vi "Range.vi"(9 "Range":dbl, 10 "Input":dbl, 11 "In Range of":dbl) -> (3 "In Range?":bool)   [LabVIEW 2014]
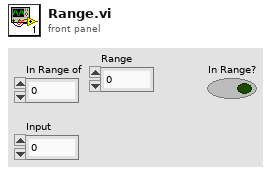
[diagram p1: front panel]
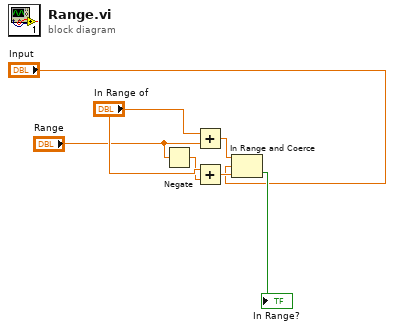
[diagram p0: block diagram]
diagram:
  n1 = Negate(x="Range") -> (-x=w5:dbl)
  n2 = Add(x="In Range of", y="Range") -> (x+y=w3:dbl)
  n3 = Add(x="In Range of", y=w5) -> (x+y=w4:dbl)
  n4 = In Range and Coerce(upper limit=w3, x="Input", lower limit=w4) -> (In Range?=→"In Range?":bool)  [unwired: 1 out]
